vi "REFPROP_ErrorConverter.vi"(8 "error in (no error)":errorcluster, 10 "Error Message":string, 11 "Error Code":i32) -> (0 "error out":errorcluster)   [LabVIEW 2021]
doc: "Converts REFPROP errors into standard error clusters."
panel:
  # "Error Converter-REFPROP.vi"
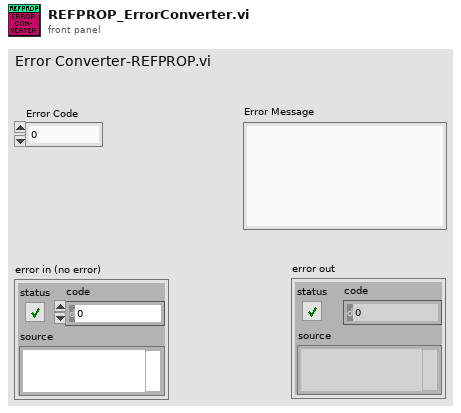
[diagram p1: front panel]
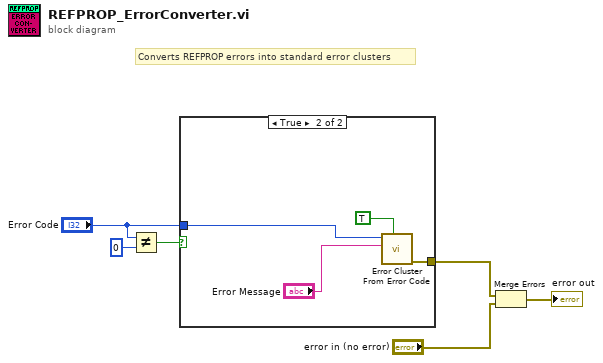
[diagram p0: block diagram]
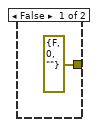
[diagram p2: hidden frame]
diagram:
  # "Converts REFPROP errors into standard error clusters"
  n1 = Not Equal?(x="Error Code", y=0) -> (x != y?=w5:bool)
  n2 = case shown="True" w5 {
    tunnel: "Error Code" -> [_ w10]
    tunnel: [errorcluster {"status"=FALSE, "code"=0, "source"=""} ("error out") w11] -> w3
    frame False {
    }
    frame True {
      n3 = call <vilib>:"Error Cluster From Error Code.vi"("show call chain? (False)"=TRUE, "error message (\"\")"="Error Message", "error code (0)"=w10) -> ("error out"=w11:errorcluster)  [unwired: 6 in]
    }
  }
  n4 = Merge Errors(w3, "error in (no error)") -> (→"error out":errorcluster)
